vi "VISCOSITY_TEMP_MONITOR.vi"(8 "DataPoints":i32=1) -> (0 "end_time":timestamp, 1 "Temp_mean":dbl format="%0.2f", 4 "ET (s)":dbl)   [LabVIEW 2019]
uses:
  CurrentRevision/5_Controls/Brookfield_type-def.ctl
  <vilib>/Instr/_visa.llb/VISA Flush IO Buffer Mask.ctl
  <vilib>/Utility/error.llb/DialogType.ctl
  <vilib>/Analysis/NI_AALBase.lvlib
panel:
  out "log_string":string
  out "start_time":timestamp
  out "Coefficient of VariationT":dbl
  out "Loop Tracker":T1[](array[typedef])
  out "ReconnectAttempts":i32
  out "TempArray":dbl[](array[numeric])
  out "error out":errorcluster
  out "Enum":T1
  out "temp":dbl
  out "Control Circuitry Enabled":bool
  out "Motor On":bool
  out "Motor Stopped":bool
  out "Auto-zero Complete":bool
  out "Motor Circuit Error":bool
  out "Diagnostics Error":bool
  out "Invalid Command Received":bool
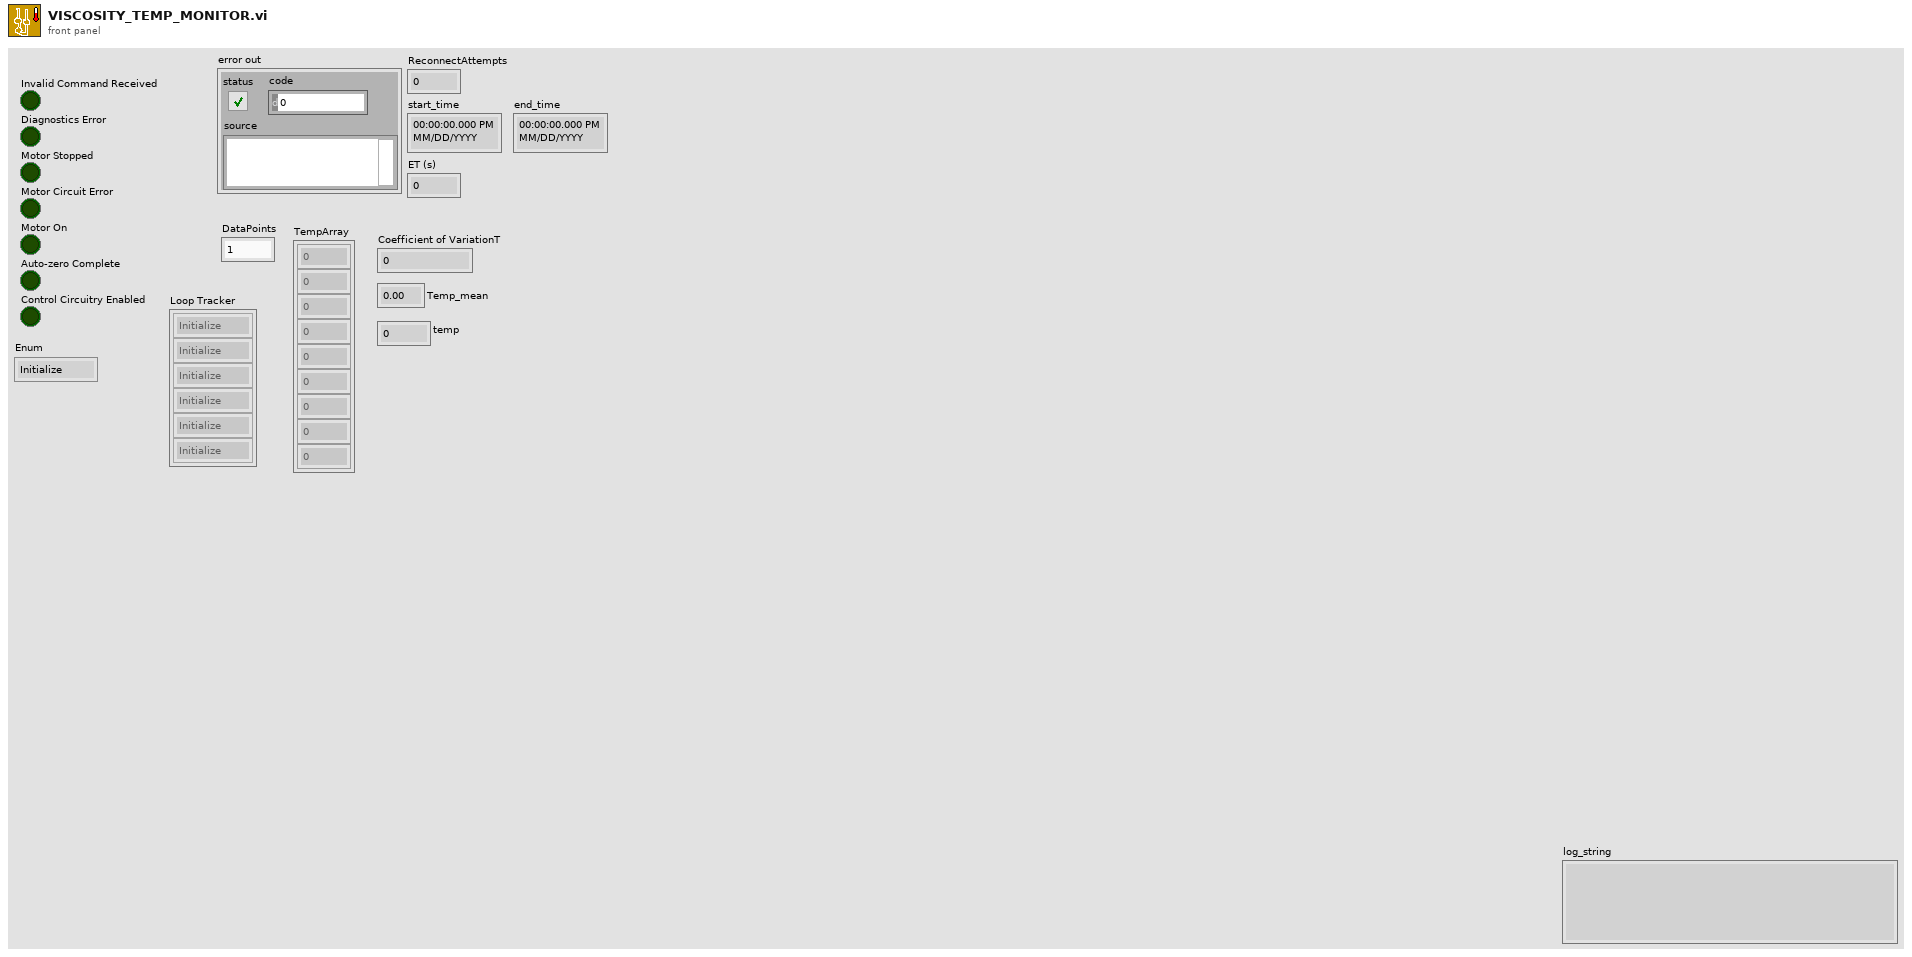
[diagram p1: front panel]
types:
  T1 = typedef "Brookfield_type-def.ctl" = enum16{"Initialize", "Enable", "Ready", "Zero", "Set Speed", "Read", "Stop Motor", "Error", "Disconnect"}
  T2 = enum16{"open", "replace", "create", "open or create", "replace or create", "replace or create with confirmation"}
  T3 = typedef "VISA Flush IO Buffer Mask.ctl" = u16
  T4 = typedef "DialogType.ctl" = u16
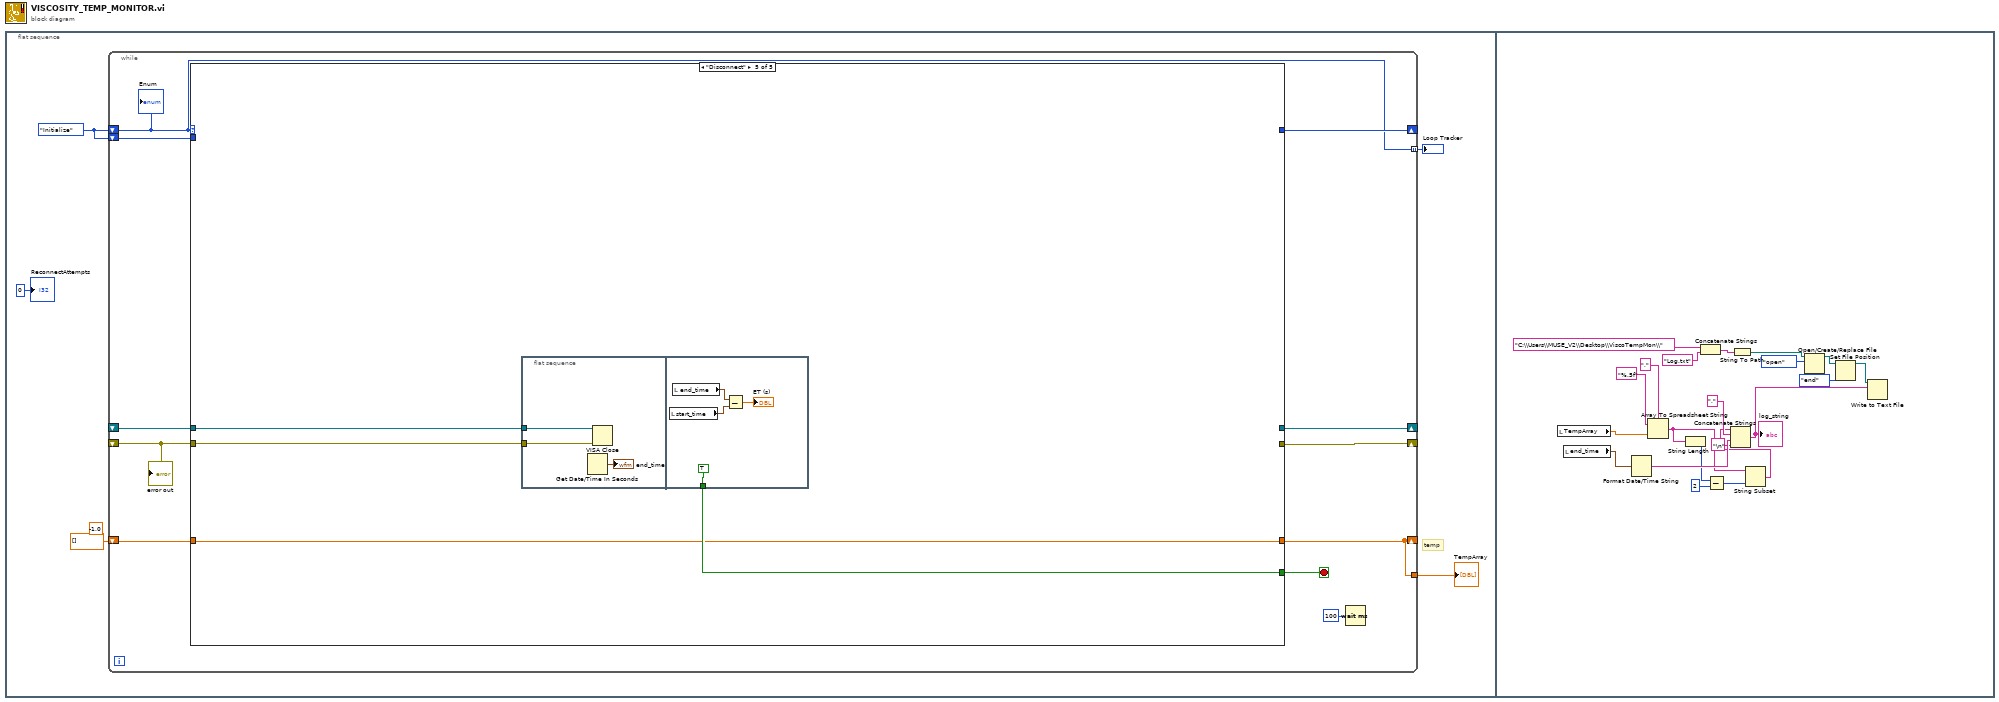
[diagram p0: block diagram]
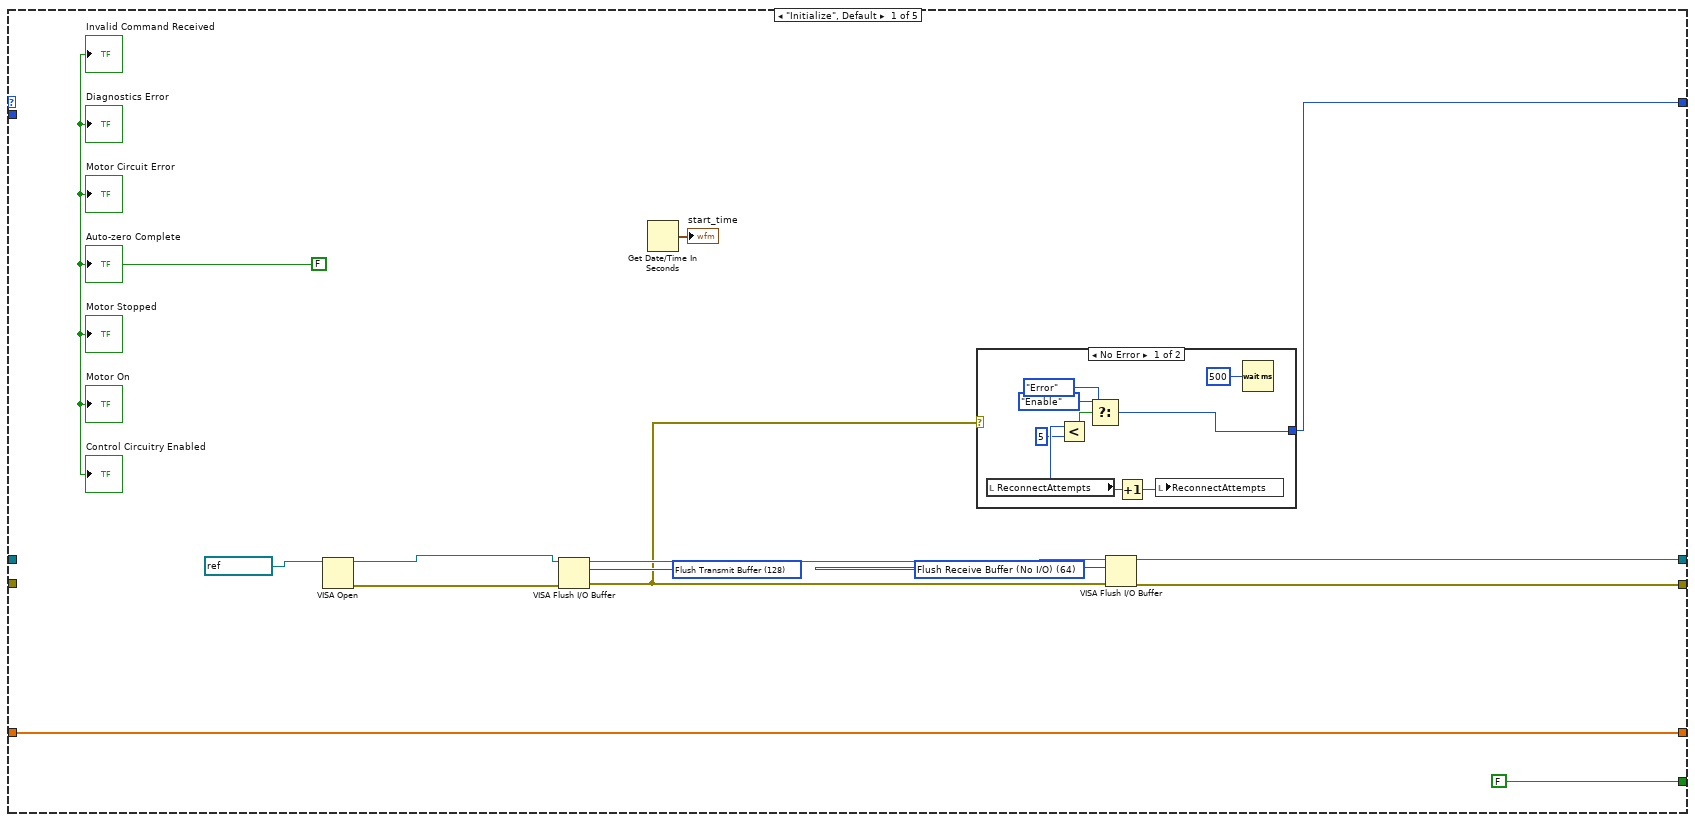
[diagram p2: hidden frame]
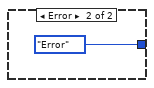
[diagram p3: hidden frame]
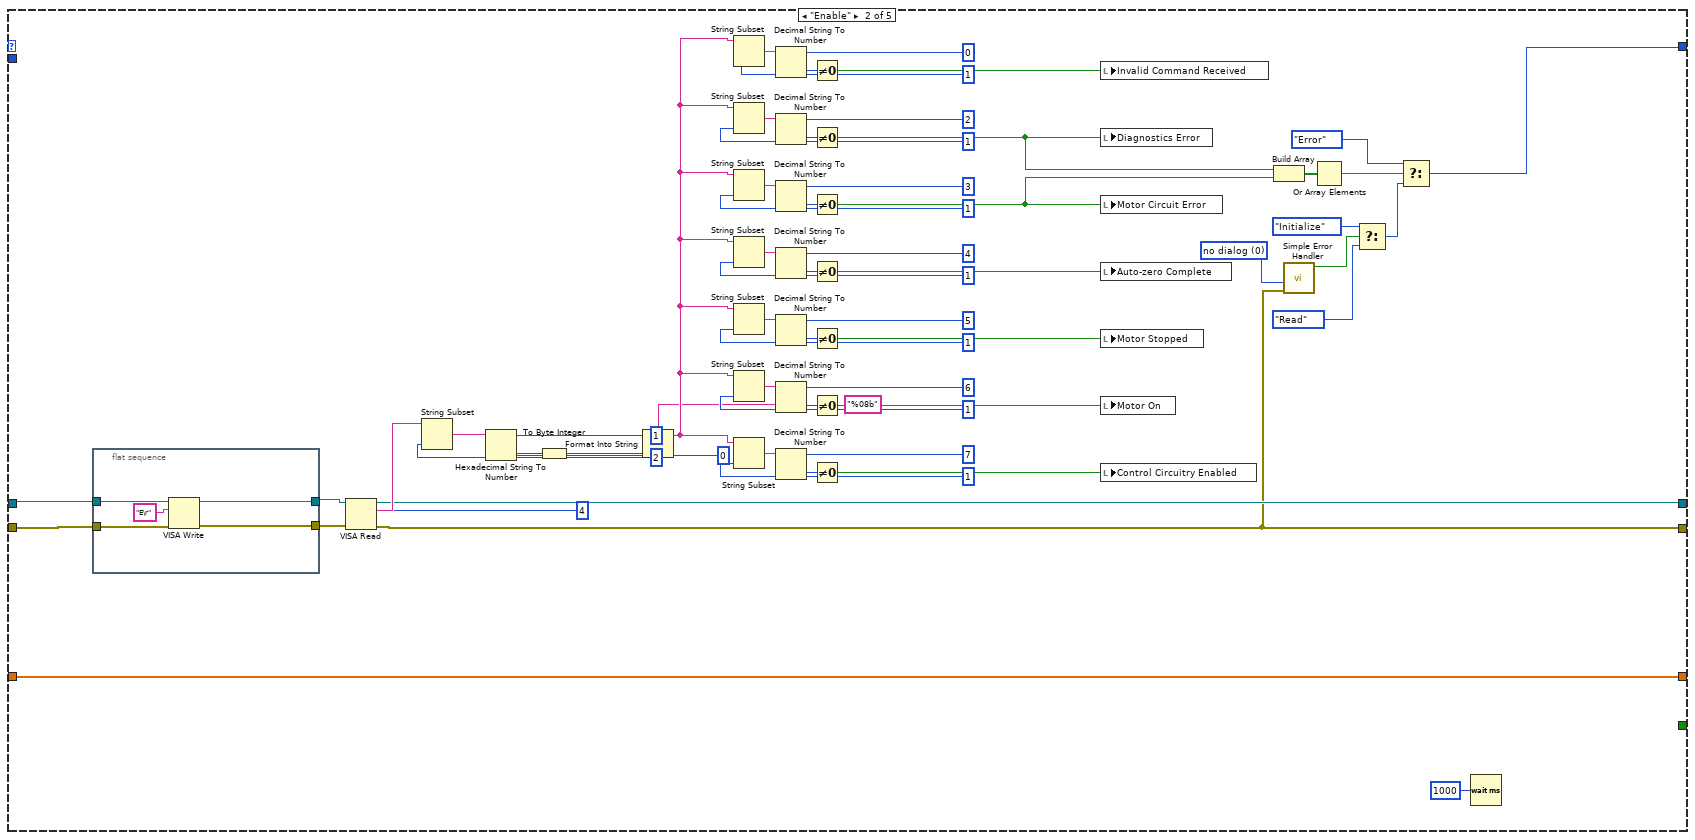
[diagram p4: hidden frame]
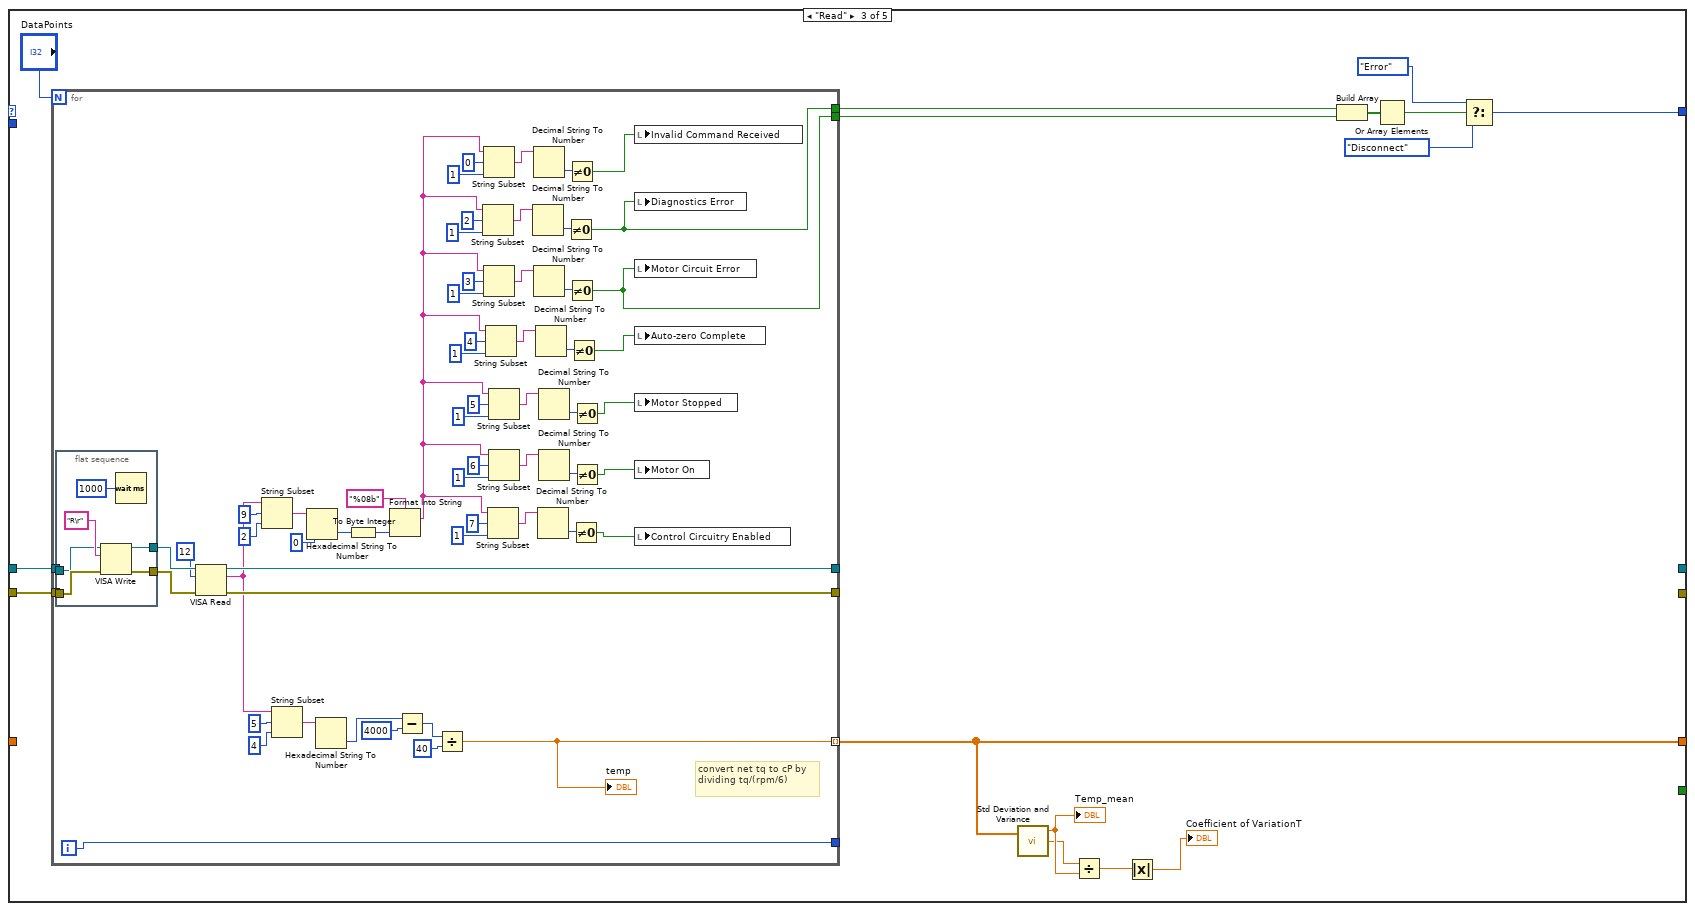
[diagram p5: hidden frame]
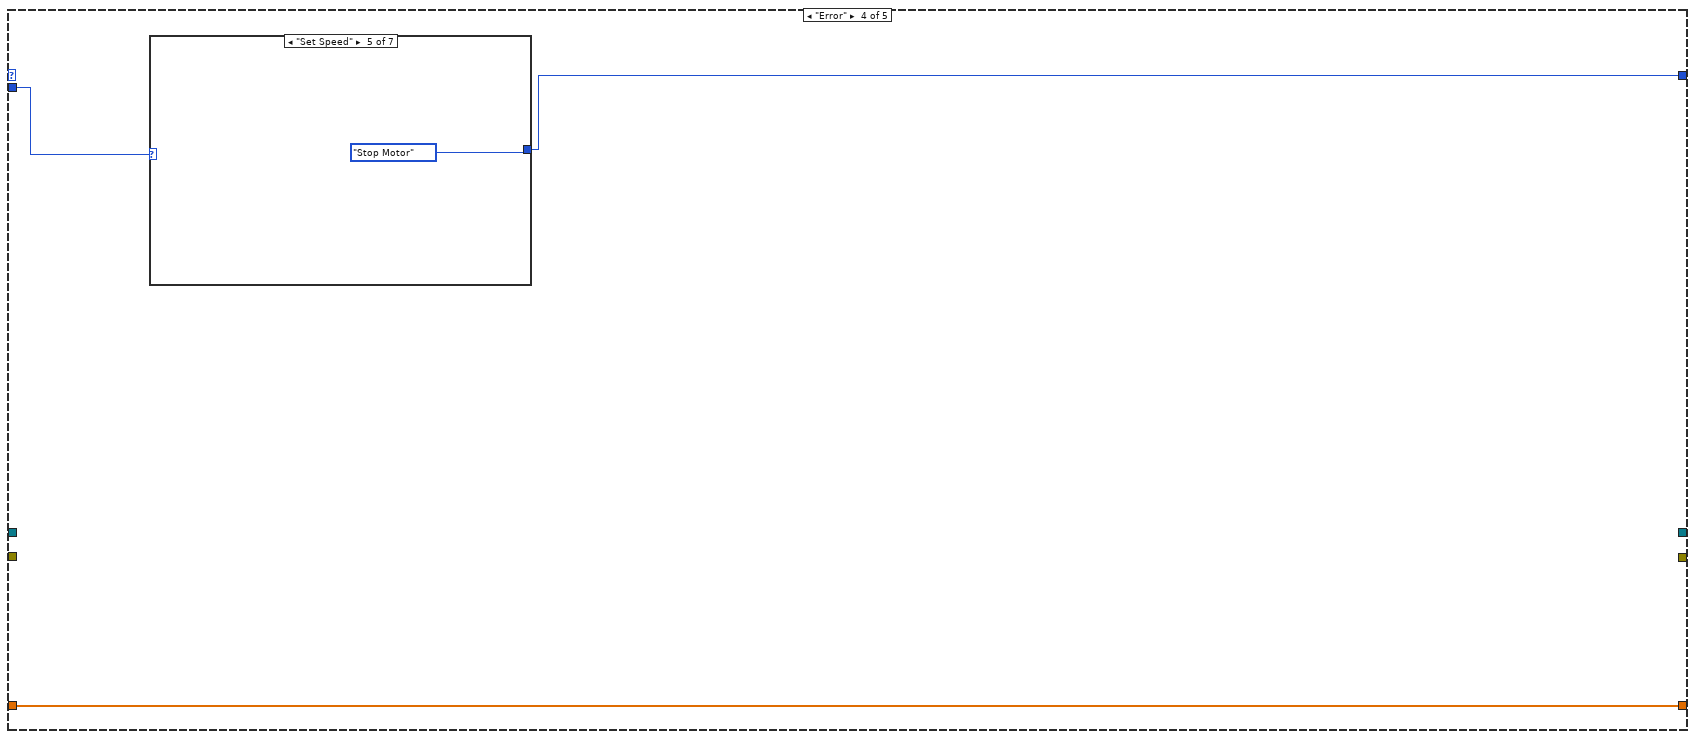
[diagram p6: hidden frame]
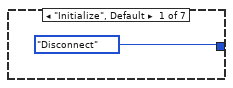
[diagram p7: hidden frame]
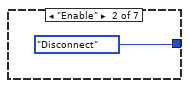
[diagram p8: hidden frame]
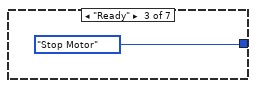
[diagram p9: hidden frame]
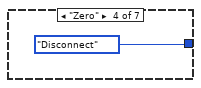
[diagram p10: hidden frame]
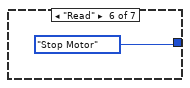
[diagram p11: hidden frame]
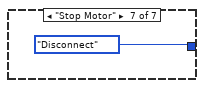
[diagram p12: hidden frame]
diagram:
  n1 = flat-sequence {
    frame #0 {
      (unwired) -1.0
      w5 = Brookfield_type-def."Initialize"
      # "temp"
      n2 = while {
        shift-right: [w7] -> _
        shift-left: w5 -> [w6]
        shift-right: [w16] -> _
        shift-left: _ -> [w14]
        shift-right: [w15] -> _
        shift-left: _ -> [w13]
        shift-right: [w8] -> _
        shift-left: dbl[] [] -> [w10]
        shift-left: w5 -> [w11]
        tunnel: [w8] -> w3
        tunnel: [w6] -> w1 mode=indexing
        stop <- w12 stop-if-true
        n3 = case shown="\"Disconnect\"" w6 {
          tunnel: [w19 w56 _ _ _] -> w16
          tunnel: [w18 w41 _ _ _] -> w15
          tunnel: w14 -> [_ w101 w114 _ w201]
          tunnel: w13 -> [_ w100 w115 _ w200]
          tunnel: [FALSE _ _ _ w199] -> w12
          tunnel: [w27 w50 w118 w190 _] -> w7
          tunnel: [w26 w49 w108 w189 w198] -> w8
          tunnel: w11 -> [_ _ _ w188 _]
          tunnel: w10 -> [w26 w49 _ w189 w198]
          frame "Initialize", Default {
            w20 = T3 64 items=["Flush Receive Buffer"=16, "Write Transmit Buffer to Device"=32, "Flush Receive Buffer (No I/O)"=64, "Flush Transmit Buffer"=128] ("Mask")
            w23 = T3 128 items=["Flush Receive Buffer"=16, "Write Transmit Buffer to Device"=32, "Flush Receive Buffer (No I/O)"=64, "Flush Transmit Buffer"=128] ("Mask")
            w29 = FALSE
            n4 = VISA Open(VISA resource name=refnum<visa-resource-name> "COM10" ("Conductivity Port")) -> (VISA resource name=w24:refnum<visa-resource-name>, error out=w25:errorcluster)  [unwired: 4 in]
            n5 = VISA Flush I/O Buffer(VISA resource name=w24, mask (16)=w23, error in (no error)=w25) -> (VISA resource name out=w22:refnum<visa-resource-name>, error out=w21:errorcluster)
            n6 = Get Date/Time In Seconds() -> (seconds since 1Jan1904=→"start_time":timestamp)
            n7 = case shown="No Error" w21 {
              tunnel: [w33 Brookfield_type-def."Error"] -> w27
              frame No Error {
                n8 = local read "ReconnectAttempts"() -> (w36:i32)
                n9 = Less?(x=w36, y=5) -> (x < y?=w34:bool)
                n10 = Select(t=Brookfield_type-def."Enable", s=w34, f=Brookfield_type-def."Error") -> (s? t:f=w33:T1)
                n11 = Increment(x=w36) -> (x+1=w37:i32)
                n12 = local write "ReconnectAttempts"(w37) -> ()
                n13 = Wait (ms)(milliseconds to wait=u32 500) -> ()  [unwired: 1 out]
              }
              frame Error {
              }
            }
            n14 = VISA Flush I/O Buffer(VISA resource name=w22, mask (16)=w20, error in (no error)=w21) -> (VISA resource name out=w19:refnum<visa-resource-name>, error out=w18:errorcluster)
            "Invalid Command Received" <- w29
            "Diagnostics Error" <- w29
            "Motor Circuit Error" <- w29
            "Auto-zero Complete" <- w29
            "Motor Stopped" <- w29
            "Motor On" <- w29
            "Control Circuitry Enabled" <- w29
          }
          frame "Enable" {
            w43 = T4 0 items=["no dialog", "OK message", "continue or stop message", "OK message + warnings", "continue/stop + warnings"] ("type of dialog (OK msg:1)")
            n15 = flat-sequence {
              tunnel: w101 -> [w105]
              tunnel: w100 -> [w104]
              tunnel: [w103] -> w42
              tunnel: [w102] -> w57
              frame #0 {
                n16 = VISA Write(VISA resource name=w105, write buffer="E\r", error in (no error)=w104) -> (VISA resource name out=w102:refnum<visa-resource-name>, error out=w103:errorcluster)  [unwired: 1 out]
              }
            }
            n17 = VISA Read(VISA resource name=w57, byte count=u32 4, error in (no error)=w42) -> (VISA resource name out=w56:refnum<visa-resource-name>, read buffer=w99:string, error out=w41:errorcluster)  [unwired: 1 out]
            n18 = String Subset(string=w99, offset (0)=1, length (rest)=2 ("length (rest)")) -> (substring=w93:string)
            n19 = Hexadecimal String To Number(string=w93, default (0uL)=u32 0 ("default (0 U32)")) -> (number=w89:u32)  [unwired: 1 in, 1 out]
            n20 = To Byte Integer(number=w89) -> (8bit integer=w90:i8)
            n21 = Format Into String(format string="%08b", w90) -> (resulting string=w76:string)  [unwired: 2 in, 1 out]
            n22 = String Subset(string=w76, offset (0)=0, length (rest)=1 ("length (rest)")) -> (substring=w92:string)
            n23 = String Subset(string=w76, offset (0)=2, length (rest)=1 ("length (rest)")) -> (substring=w87:string)
            n24 = String Subset(string=w76, offset (0)=3, length (rest)=1 ("length (rest)")) -> (substring=w86:string)
            n25 = String Subset(string=w76, offset (0)=4, length (rest)=1 ("length (rest)")) -> (substring=w83:string)
            n26 = String Subset(string=w76, offset (0)=5, length (rest)=1 ("length (rest)")) -> (substring=w82:string)
            n27 = String Subset(string=w76, offset (0)=6, length (rest)=1 ("length (rest)")) -> (substring=w79:string)
            n28 = String Subset(string=w76, offset (0)=7, length (rest)=1 ("length (rest)")) -> (substring=w78:string)
            n29 = Decimal String To Number(string=w92) -> (number=w91:i32)  [unwired: 2 in, 1 out]
            n30 = Decimal String To Number(string=w87) -> (number=w88:i32)  [unwired: 2 in, 1 out]
            n31 = Decimal String To Number(string=w86) -> (number=w85:i32)  [unwired: 2 in, 1 out]
            n32 = Decimal String To Number(string=w83) -> (number=w84:i32)  [unwired: 2 in, 1 out]
            n33 = Decimal String To Number(string=w82) -> (number=w81:i32)  [unwired: 2 in, 1 out]
            n34 = Decimal String To Number(string=w79) -> (number=w80:i32)  [unwired: 2 in, 1 out]
            n35 = Decimal String To Number(string=w78) -> (number=w77:i32)  [unwired: 2 in, 1 out]
            n36 = Not Equal To 0?(x=w91) -> (x != 0?=w94:bool)
            n37 = Not Equal To 0?(x=w88) -> (x != 0?=w55:bool)
            n38 = Not Equal To 0?(x=w85) -> (x != 0?=w54:bool)
            n39 = Not Equal To 0?(x=w84) -> (x != 0?=w95:bool)
            n40 = Not Equal To 0?(x=w81) -> (x != 0?=w96:bool)
            n41 = Not Equal To 0?(x=w80) -> (x != 0?=w97:bool)
            n42 = Not Equal To 0?(x=w77) -> (x != 0?=w98:bool)
            n43 = local write "Invalid Command Received"(w94) -> ()
            n44 = local write "Diagnostics Error"(w55) -> ()
            n45 = local write "Motor Circuit Error"(w54) -> ()
            n46 = local write "Auto-zero Complete"(w95) -> ()
            n47 = local write "Motor Stopped"(w96) -> ()
            n48 = local write "Motor On"(w97) -> ()
            n49 = local write "Control Circuitry Enabled"(w98) -> ()
            n50 = Build Array(w55, w54) -> (w53:bool[])
            n51 = call <vilib>:"Simple Error Handler.vi"("type of dialog (OK msg:1)"=w43, "error in (no error)"=w41) -> ("error?"=w45:bool)  [unwired: 3 in, 4 out]
            n52 = Or Array Elements(Boolean array=w53) -> (logical OR=w52:bool)
            n53 = Select(t=Brookfield_type-def."Initialize", s=w45, f=Brookfield_type-def."Read") -> (s? t:f=w48:T1)
            n54 = Select(t=Brookfield_type-def."Error", s=w52, f=w48) -> (s? t:f=w50:T1)
            n55 = Wait (ms)(milliseconds to wait=u32 1000) -> ()  [unwired: 1 out]
          }
          frame "Read" {
            n56 = for {
              N: "DataPoints" -> [_]
              tunnel: [w181] -> _
              tunnel: [w180] -> _
              tunnel: [w179] -> w117
              tunnel: [w178] -> w116
              tunnel: [w177] -> w108 mode=indexing
              tunnel: w115 -> [w176]
              tunnel: w114 -> [w175]
              tunnel: [w122] -> _
              i -> [w122]
              # "convert net tq to cP by dividing tq/(rpm/6)"
              n57 = flat-sequence {
                tunnel: w176 -> [w186]
                tunnel: w175 -> [w184]
                tunnel: [w183] -> w174
                tunnel: [w182] -> w173
                frame #0 {
                  n58 = VISA Write(VISA resource name=w184, write buffer="R\r", error in (no error)=w186) -> (VISA resource name out=w182:refnum<visa-resource-name>, error out=w183:errorcluster)  [unwired: 1 out]
                  n59 = Wait (ms)(milliseconds to wait=u32 1000) -> ()  [unwired: 1 out]
                }
              }
              n60 = VISA Read(VISA resource name=w173, byte count=u32 12, error in (no error)=w174) -> (VISA resource name out=w181:refnum<visa-resource-name>, read buffer=w162:string, error out=w180:errorcluster)  [unwired: 1 out]
              n61 = String Subset(string=w162, offset (0)=9, length (rest)=2 ("length (rest)")) -> (substring=w161:string)
              n62 = String Subset(string=w162, offset (0)=5, length (rest)=4 ("length (rest)")) -> (substring=w168:string)
              n63 = Hexadecimal String To Number(string=w161, default (0uL)=u32 0 ("default (0 U32)")) -> (number=w153:u32)  [unwired: 1 in, 1 out]
              n64 = Hexadecimal String To Number(string=w168) -> (number=w167:u32)  [unwired: 2 in, 1 out]
              n65 = To Byte Integer(number=w153) -> (8bit integer=w154:i8)
              n66 = Format Into String(format string="%08b", w154) -> (resulting string=w128:string)  [unwired: 2 in, 1 out]
              n67 = Subtract(x=w167, y=u32 4000) -> (x-y=w165:u32)
              n68 = Divide(x=w165, y=u32 40) -> (x/y=w177:dbl)
              "temp" <- w177
              n69 = String Subset(string=w128, offset (0)=2, length (rest)=1 ("length (rest)")) -> (substring=w151:string)
              n70 = String Subset(string=w128, offset (0)=0, length (rest)=1 ("length (rest)")) -> (substring=w157:string)
              n71 = String Subset(string=w128, offset (0)=3, length (rest)=1 ("length (rest)")) -> (substring=w146:string)
              n72 = String Subset(string=w128, offset (0)=4, length (rest)=1 ("length (rest)")) -> (substring=w143:string)
              n73 = String Subset(string=w128, offset (0)=7, length (rest)=1 ("length (rest)")) -> (substring=w130:string)
              n74 = String Subset(string=w128, offset (0)=5, length (rest)=1 ("length (rest)")) -> (substring=w138:string)
              n75 = String Subset(string=w128, offset (0)=6, length (rest)=1 ("length (rest)")) -> (substring=w135:string)
              n76 = Decimal String To Number(string=w151) -> (number=w152:i32)  [unwired: 2 in, 1 out]
              n77 = Decimal String To Number(string=w157) -> (number=w156:i32)  [unwired: 2 in, 1 out]
              n78 = Decimal String To Number(string=w146) -> (number=w145:i32)  [unwired: 2 in, 1 out]
              n79 = Decimal String To Number(string=w143) -> (number=w144:i32)  [unwired: 2 in, 1 out]
              n80 = Decimal String To Number(string=w130) -> (number=w129:i32)  [unwired: 2 in, 1 out]
              n81 = Decimal String To Number(string=w138) -> (number=w137:i32)  [unwired: 2 in, 1 out]
              n82 = Decimal String To Number(string=w135) -> (number=w136:i32)  [unwired: 2 in, 1 out]
              n83 = Not Equal To 0?(x=w152) -> (x != 0?=w179:bool)
              n84 = Not Equal To 0?(x=w156) -> (x != 0?=w123:bool)
              n85 = Not Equal To 0?(x=w145) -> (x != 0?=w178:bool)
              n86 = Not Equal To 0?(x=w144) -> (x != 0?=w124:bool)
              n87 = Not Equal To 0?(x=w129) -> (x != 0?=w127:bool)
              n88 = Not Equal To 0?(x=w137) -> (x != 0?=w125:bool)
              n89 = Not Equal To 0?(x=w136) -> (x != 0?=w126:bool)
              n90 = local write "Invalid Command Received"(w123) -> ()
              n91 = local write "Diagnostics Error"(w179) -> ()
              n92 = local write "Motor Circuit Error"(w178) -> ()
              n93 = local write "Auto-zero Complete"(w124) -> ()
              n94 = local write "Motor Stopped"(w125) -> ()
              n95 = local write "Motor On"(w126) -> ()
              n96 = local write "Control Circuitry Enabled"(w127) -> ()
            }
            n97 = call <vilib>:"Std Deviation and Variance.vi"("X"=w108) -> ("mean"=w110:dbl, "standard deviation"=w109:dbl)  [unwired: 1 in, 1 out]
            "Temp_mean" <- w110
            n98 = Divide(x=w109, y=w110) -> (x/y=w111:dbl)
            n99 = Absolute Value(x=w111) -> (abs(x)=→"Coefficient of VariationT":dbl)
            n100 = Build Array(w117, w116) -> (w119:bool[])
            n101 = Or Array Elements(Boolean array=w119) -> (logical OR=w121:bool)
            n102 = Select(t=Brookfield_type-def."Error", s=w121, f=Brookfield_type-def."Disconnect") -> (s? t:f=w118:T1)
          }
          frame "Error" {
            n103 = case shown="\"Set Speed\"" w188 {
              tunnel: [Brookfield_type-def."Disconnect" Brookfield_type-def."Disconnect" Brookfield_type-def."Stop Motor" Brookfield_type-def."Disconnect" Brookfield_type-def."Stop Motor" Brookfield_type-def."Stop Motor" Brookfield_type-def."Disconnect"] -> w190
              frame "Initialize", Default {
              }
              frame "Enable" {
              }
              frame "Ready" {
              }
              frame "Zero" {
              }
              frame "Set Speed" {
              }
              frame "Read" {
              }
              frame "Stop Motor" {
              }
            }
          }
          frame "Disconnect" {
            n104 = flat-sequence {
              tunnel: w201 -> [w204]
              tunnel: w200 -> [w203]
              tunnel: [TRUE] -> w199
              frame #0 {
                n105 = Get Date/Time In Seconds() -> (seconds since 1Jan1904=→"end_time":timestamp)
                n106 = VISA Close(VISA resource name=w204, error in (no error)=w203) -> ()  [unwired: 1 out]
              }
              frame #1 {
                n107 = local read "start_time"() -> (w206:timestamp)
                n108 = local read "end_time"() -> (w207:timestamp)
                n109 = Subtract(x=w207, y=w206) -> (x-y=→"ET (s)":dbl)
              }
            }
          }
        }
        n110 = Wait (ms)(milliseconds to wait=u32 100) -> ()  [unwired: 1 out]
        "Enum" <- w6
        "error out" <- w13
      }
      "TempArray" <- w3
      "Loop Tracker" <- w1
      "ReconnectAttempts" <- 0
    }
    frame #1 {
      n111 = local read "TempArray"() -> (w220:dbl[])
      n112 = local read "end_time"() -> (w219:timestamp)
      n113 = Format Date/Time String(seconds (now)=w219) -> (date/time string=w218:string)  [unwired: 2 in]
      n114 = Array To Spreadsheet String(delimiter (Tab)=",", array=w220, 3:"%.5f" ("format (%.3f)")) -> (spreadsheet string=w214:string)
      n115 = String Length(string=w214) -> (length=w211:i32)
      n116 = Concatenate Strings("C:\\Users\\MUSE_V2\\Desktop\\ViscoTempMon\\", "Log.txt" ("string")) -> (w228:string)
      n117 = Subtract(x=w211, y=2) -> (x-y=w209:i32)
      n118 = String To Path(string=w228) -> (path=w227:path)
      n119 = String Subset(string=w214, length (rest)=w209) -> (substring=w213:string)  [unwired: 1 in]
      n120 = Concatenate Strings(w213, ",", w218, "\n" ("string")) -> (w224:string)
      "log_string" <- w224
      n121 = Open/Create/Replace File(file path (use dialog)=w227, operation (0:open)=T2."open") -> (refnum out=w217:refnum<file>)  [unwired: 4 in, 2 out]
      n122 = Set File Position(refnum=w217, from (0:start)=enum16{"start", "end", "current"}."end") -> (refnum out=w216:refnum<file>)  [unwired: 2 in, 1 out]
      n123 = Write to Text File(file (use dialog)=w216, text=w224) -> ()  [unwired: 2 in, 3 out]
    }
  }
